vi "Test Default Text Comparator.vi"(11 "Test Case In":refnum<class "Comparator Tests.lvclass">) -> (0 "error out":errorcluster, 3 "Test Case Out":refnum<class "Comparator Tests.lvclass">)   [LabVIEW 2020, in "Comparator Tests.lvclass"]
uses:
  Comparator Tests.lvclass
  C:/Program Files/National Instruments/LabVIEW 2026/vi.lib/Astemes/LUnit/Test Case.lvclass
  Source/Approval Tests/Text Comparator/Text Comparator.lvclass
  <vilib>/Astemes/LUnit/Test Case.lvclass/Test Case.ctl
  <vilib>/Astemes/LUnit/Core/LUnit Test Case/Private/Append Fail Result.vi
  <vilib>/Astemes/LUnit/Core/LUnit Test Case/Private/Append Pass Result.vi
  <vilib>/Astemes/LUnit/Core/LUnit Test Case/Private/Run In UI.vi
  <vilib>/Utility/error.llb/Clear Errors.vi
  <vilib>/Astemes/LUnit/Test Case.lvclass
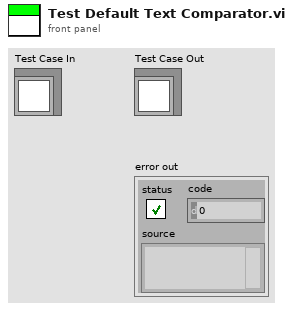
[diagram p1: front panel]
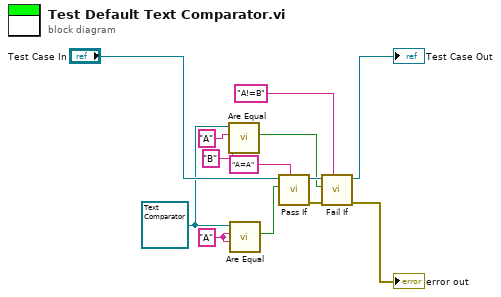
[diagram p0: block diagram]
diagram:
  w4 = "A" ("Approved Text")
  w6 = refnum<class "Text Comparator.lvclass"> refnum ("Approval Tests:Text Comparator")
  n1 = call-dynamic "Are Equal.vi"("Received Text"="B", "Approved Text"="A", "Text Comparator in"=w6) -> ("Are Equal?"=w5:bool)  [unwired: 6 in, 2 out]
  n2 = call-dynamic "Are Equal.vi"("Received Text"=w4, "Approved Text"=w4, "Text Comparator in"=w6) -> ("Are Equal?"=w10:bool)  [unwired: 6 in, 2 out]
  n3 = call <vilib>:"Pass If.vi"("Description"="A=A", "Pass?"=w10, "LUnit Test Case In"="Test Case In") -> ("error out"=w13:errorcluster, "LUnit Test Case Out"=w9:refnum<class "Comparator Tests.lvclass">)  [unwired: 7 in]
  n4 = call <vilib>:"Fail If.vi"("Description"="A!=B", "error in (no error)"=w13, "Fail?"=w5, "LUnit Test Case In"=w9) -> ("error out"=→"error out":errorcluster, "LUnit Test Case Out"=→"Test Case Out":refnum<class "Comparator Tests.lvclass">)  [unwired: 6 in]
